vi "Manual with LIDAR localisation - logging.vi"() -> ()   [LabVIEW 2017]
uses:
  enc based vel calc FGVs/Action Items.ctl
  <instrlib>/Hokuyo URG Series/Public/Initialize-cRIO-USB.vi
  <vilib>/functionblocks/Counter/Elapsed Timer/Elapsed Timer.vi
  <vilib>/functionblocks/FB Core/FB Core.xnode
  <instrlib>/Hokuyo URG Series/Hokuyo URG Series.lvlib
  <vilib>/functionblocks/NI_FunctionBlock Libraries.lvlib
panel:
  out "desired movement angle":dbl
  in  "Desired orientation":dbl
  in  "Orientation for max rotation":dbl=30.0
  out "Localisation dt (ms)":i32
  out "dy":dbl
  out "dx":dbl
  in  "Delay (s)":dbl
  out "Remaining delay":dbl
  out "y ref":dbl
  out "y":dbl
  out "x ref":dbl
  out "x":dbl
  in  "Min orientation for rotation":dbl=5.0
  in  "Rot min abs spd":dbl=0.5
  in  "Motor Stop (esc)":bool
  in  "Initial position":cluster{"X":dbl, "Y":dbl}={"X"=250.0, "Y"=1650.0}
  in  "Right":bool
  in  "Left":bool
  in  "Down":bool
  in  "Up":bool
  in  "Protocol":u32(ring)=2 items=["Convert to Latest", "SCIP 1.1", "SCIP 2.0"]
  in  "ID Query?":bool=TRUE
  in  "Checksum":bool
  in  "Stop":bool
  out "XY Graph 6m max":cluster{"Y":dbl[], "Y":dbl[]}[](graph)
  in  "Rot spd multiplier":dbl=2.0
  in  "error in":errorcluster
  in  "Trans spd multiplier":dbl=2.0
  in  "PID gains":T1={"proportional gain (Kc)"=0.01, "integral time (Ti, min)"=0.003, "derivative time (Td, min)"=0.0} {"derivative time (Td, min)" format="%.6f"; "integral time (Ti, min)" format="%.6f"; "proportional gain (Kc)" format="%.6f"}
  # "P:  Higher the number, higher the abrupt change\nI: Higher the number, the less it tries to overshoot"
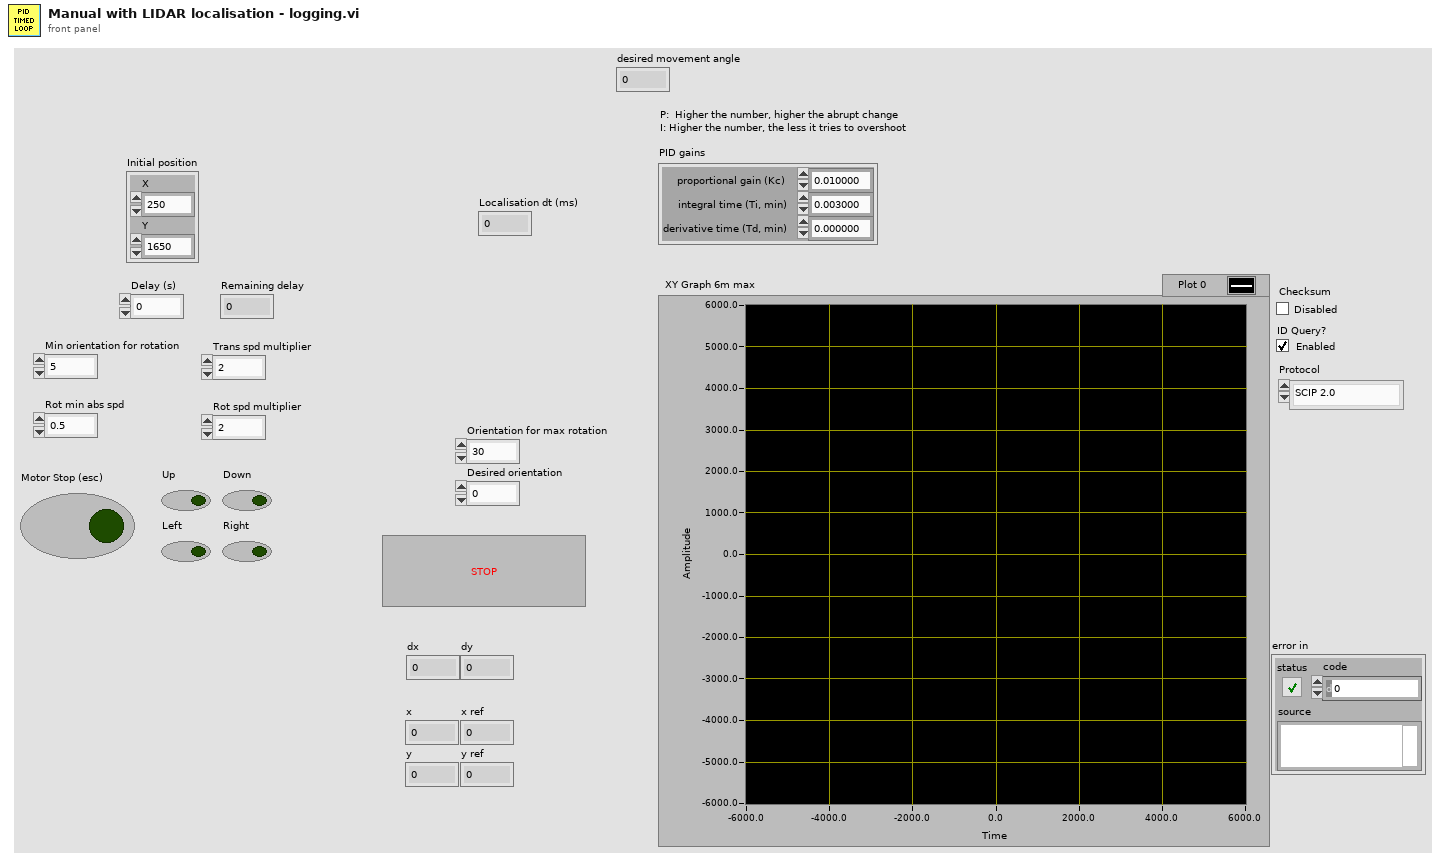
[diagram p1: front panel]
types:
  T1 = cluster{"proportional gain (Kc)":dbl, "integral time (Ti, min)":dbl, "derivative time (Td, min)":dbl}
  T2 = typedef "Action Items.ctl" = enum16{"Initialize", "Read"}
  T3 = enum16{"Stop / None", "Forward", "Backward", "Left", "Right", "Manual"}
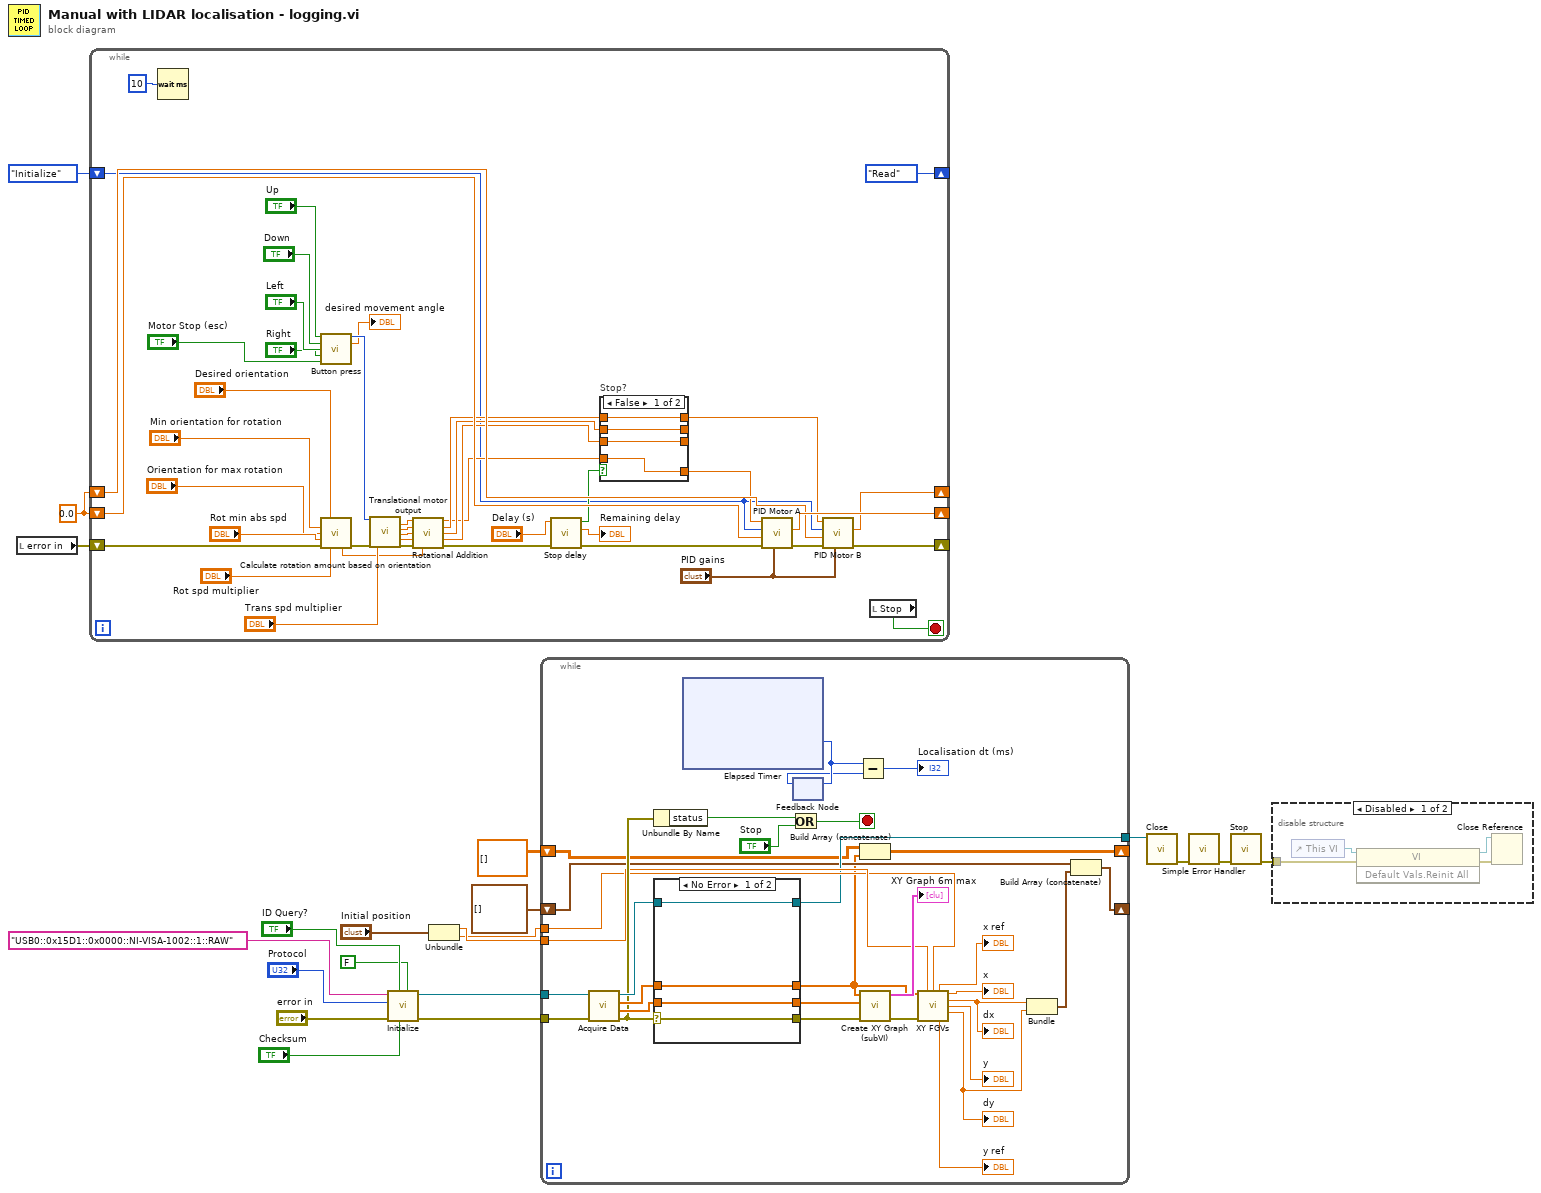
[diagram p0: block diagram]
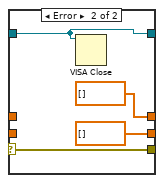
[diagram p2: hidden frame]
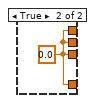
[diagram p3: hidden frame]
diagram:
  w14 = 0.0 ("output")
  n1 = local read "error in"() -> (w1:errorcluster)
  n2 = while {
    shift-right: [w61] -> _
    shift-left: w14 -> [w63]
    shift-right: [Action_Items."Read" ("Action")] -> _
    shift-left: Action_Items."Initialize" ("Action") -> [w31]
    shift-right: [w59] -> _
    shift-left: w14 -> [w58]
    shift-right: [w22] -> _
    shift-left: w1 -> [w21]
    stop <- w28 stop-if-true
    n3 = Wait (ms)(milliseconds to wait=u32 10) -> ()  [unwired: 1 out]
    n4 = call "Button press.vi"("Up"="Up", "Down"="Down", "Left"="Left", "Right"="Right", "Stop"="Motor Stop (esc)") -> ("Command"=w50:T3, "angle"=→"desired movement angle":dbl)  [unwired: 9 in]
    n5 = call "Calculate rotation amount based on orientation.vi"("Desired orientation"="Desired orientation", "Min orientation for rotation"="Min orientation for rotation", "Orientation for max rotation"="Orientation for max rotation", "Rot min abs spd"="Rot min abs spd", "error in"=w21, "Rot spd multiplier"="Rot spd multiplier") -> ("Rot spd out"=w43:dbl, "error out"=w24:errorcluster)  [unwired: 6 in, 2 out]
    n6 = call "Translational motor output.vi"("Command"=w50, "error in"=w24, "Trans spd multiplier"="Trans spd multiplier") -> ("motor 1 out"=w52:dbl, "motor 2 out"=w53:dbl, "motor 3 out"=w54:dbl, "motor 4 out"=w55:dbl, "error out"=w56:errorcluster)  [unwired: 12 in]
    n7 = call "Rotational Addition.vi"("Motor 1 in"=w52, "Motor 2 in"=w53, "Motor 3 in"=w54, "Motor 4 in"=w55, "error in"=w56, "Rot spd multiplier"=w43) -> ("Motor 1 out"=w38:dbl, "Motor 2 out"=w40:dbl, "Motor 3 out"=w41:dbl, "Motor 4 out"=w42:dbl, "error out"=w35:errorcluster)  [unwired: 5 in]
    n8 = call "Stop delay.vi"("error in (no error)"=w35, "Delay (s)"="Delay (s)") -> ("error out"=w34:errorcluster, "Remaining delay"=→"Remaining delay":dbl, "Stop?"=w36:bool)  [unwired: 7 in]
    n9 = case "Stop?" shown="False" w36 {
      tunnel: w42 -> [w67 _]
      tunnel: [w67 w68] -> _
      tunnel: w41 -> [w66 _]
      tunnel: [w66 w68] -> _
      tunnel: w40 -> [w65 _]
      tunnel: [w65 w68] -> w39
      tunnel: w38 -> [w64 _]
      tunnel: [w64 w68] -> w37
      frame False {
      }
      frame True {
        w68 = 0.0 ("Motor 3 out")
      }
    }
    n10 = call "PID Motor A.vi"("PID gains"="PID gains", "error in (no error)"=w34, "input"=w63, "dt in (ms)"=w31, "Setpoint A0"=w37) -> ("error out"=w60:errorcluster, "output"=w61:dbl)  [unwired: 1 in, 4 out]
    n11 = call "PID Motor B.vi"("PID gains"="PID gains", "error in (no error)"=w60, "input"=w58, "dt in (ms)"=w31, "Setpoint B0"=w39) -> ("error out"=w22:errorcluster, "output"=w59:dbl)  [unwired: 1 in, 4 out]
    n12 = local read "Stop"() -> (w28:bool)
  }
  n13 = call-poly <instrlib>:"Initialize.vi"("Reset? (F: No)"=FALSE ("Reset Instrument (Disabled)"), "Checksum (Disabled)"="Checksum", "ID Query? (Enabled)"="ID Query?", "error in (no error)"="error in", "Protocol (2: SCIP 2.0)"="Protocol", "VISA resource name"="USB0::0x15D1::0x0000::NI-VISA-1002::1::RAW") -> ("error out"=w10:errorcluster, "VISA resource name out"=w9:refnum<visa-resource-name>)  [unwired: 4 in]
  n14 = Unbundle("Initial position") -> ("X"=w13:dbl, "Y"=w12:dbl)
  n15 = while {
    tunnel: w13 -> [w84]
    tunnel: w12 -> [w83]
    tunnel: w10 -> [w80]
    tunnel: w9 -> [w79]
    tunnel: [w78] -> w4
    shift-right: [w74] -> _
    shift-left: dbl[][] [] -> [w73]
    shift-right: [w71] -> _
    shift-left: cluster{"dx":dbl, "dy":dbl}[] [] -> [w70]
    stop <- w81 stop-if-true
    n16 = call <instrlib>:"Acquire Data.vi"("error in (no error)"=w80, "VISA resource name"=w79) -> ("error out"=w88:errorcluster, "Direction"=w89:dbl[], "Magnitude"=w92:dbl[], "VISA resource name out"=w90:refnum<visa-resource-name>)  [unwired: 6 in]
    n17 = Unbundle By Name(w88) -> ("status"=w91:bool)
    n18 = case shown="No Error" w88 {
      selector: w88 -> [w136 w143]
      tunnel: [w136 w143] -> w85
      tunnel: w90 -> [w139 w142]
      tunnel: [w139 w142] -> w78
      tunnel: w92 -> [w138 _]
      tunnel: w89 -> [w137 _]
      tunnel: [w138 dbl[] [] ("Magnitude")] -> w69
      tunnel: [w137 dbl[] [] ("Direction")] -> w86
      frame No Error {
      }
      frame Error {
        n19 = VISA Close(VISA resource name=w142) -> ()  [unwired: 1 in, 1 out]
      }
    }
    n20 = xnode "Elapsed Timer"() -> ("elapsed time (ms)"=w77:i32)  [unwired: 3 in, 1 out]
    n21 = Or(x=w91, y="Stop") -> (x .or. y?=w81:bool)
    n22 = feedback-in #1(w77) -> ()
    n23 = feedback #1() -> (w76:i32)  [unwired: 1 in]
    n24 = Subtract(x=w77, y=w76) -> (x-y=→"Localisation dt (ms)":i32)
    n25 = Build Array (concatenate)(w73, w69) -> (w74:dbl[][])
    n26 = call "Create XY Graph (subVI).vi"("error in"=w85, "Direction"=w86, "Magnitude"=w69) -> ("error out"=w93:errorcluster, "XY Graph"=→"XY Graph 6m max":cluster{"Y":dbl[], "Y":dbl[]}[])  [unwired: 6 in, 1 out]
    n27 = call "XY FGVs.vi"("LIDAR Mag"=w69, "x init"=w84, "y init"=w83, "error in (no error)"=w93) -> ("x ref"=→"x ref":dbl, "x"=→"x":dbl, "dx"=w98:dbl, "y"=→"y":dbl, "dy"=w99:dbl, "y ref"=→"y ref":dbl)  [unwired: 5 in, 1 out]
    "dx" <- w98
    "dy" <- w99
    n28 = Bundle("dx"=w98, "dy"=w99) -> (w72:cluster{"dx":dbl, "dy":dbl})  [unwired: 1 in]
    n29 = Build Array (concatenate)(w70, w72) -> (w71:cluster{"dx":dbl, "dy":dbl}[])
  }
  n30 = call <instrlib>:"Close.vi"("VISA resource name"=w4) -> ("error out"=w6:errorcluster)  [unwired: 10 in]
  n31 = call <vilib>:"Simple Error Handler.vi"("error in (no error)"=w6) -> ("error out"=w5:errorcluster)  [unwired: 4 in, 4 out]
  n32 = call "Stop.vi"("error in (no error)"=w5) -> ("OG error out"=w7:errorcluster)  [unwired: 9 in, 1 out]
  n33 = disable-structure shown="Disabled" {
    disable-tunnel: w7 -> [w144 _]
    frame Disabled {
      n34 = control-ref of="This VI"() -> (w147:refnum<vi>)
      n35 = invoke class="VI" method="Default Vals.Reinit All"(reference=w147, error in=w144) -> (reference out=w146:refnum<vi>, error out=w145:errorcluster)  [unwired: 1 in, 1 out]
      n36 = Close Reference(reference=w146, error in (no error)=w145) -> ()  [unwired: 1 out]
    }
    frame Enabled {
    }
  }
